vi "CfgManager.Text--ForceSave.vi"() -> ()   [LabVIEW 2013]
uses:
  source/Manager.Text/ConfigManager.Text.lvclass
  source/Manager/Decompose KVPs.vi
  source/Manager/Write.vi
  source/Manager/ConfigManager.lvclass
panel:
  out "Keys":string[](array[string])
  out "error out":errorcluster
  out "filepath":path
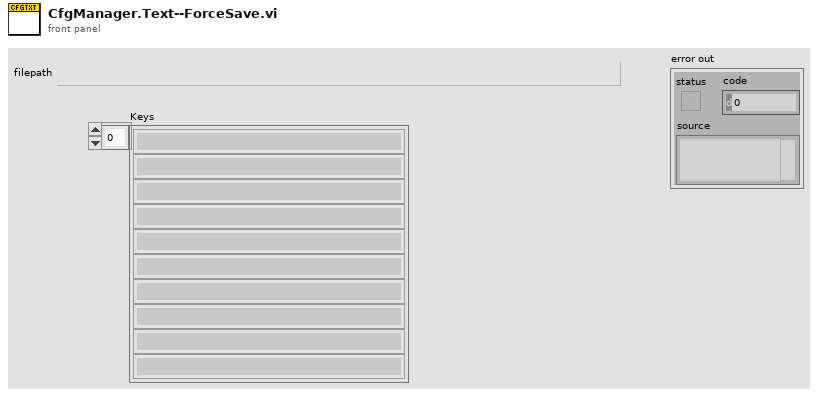
[diagram p1: front panel]
types:
  T1 = cluster{"String":string, "Numeric":dbl, "Boolean":bool}
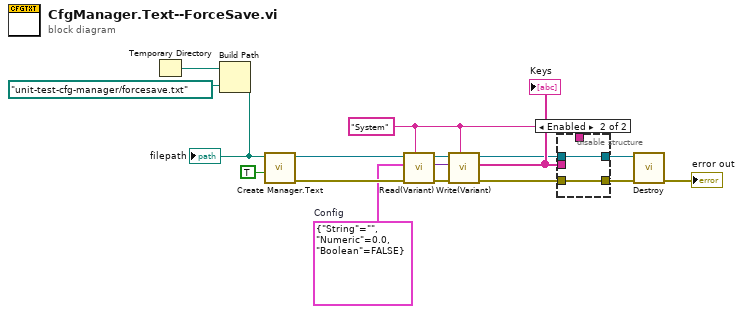
[diagram p0: block diagram]
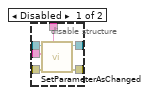
[diagram p2: hidden frame]
diagram:
  w5 = "System" ("Qualified Name")
  w10 = T1 {"String"="", "Numeric"=0.0, "Boolean"=FALSE}  # Config
  n1 = Temporary Directory() -> (w16:path)
  n2 = Build Path(base path=w16, name or relative path=path "unit-test-cfg-manager/forcesave.txt" ("filepath 2")) -> (appended path=w14:path)
  "filepath" <- w14
  n3 = call "Create Manager.Text.vi"("Create if Non Existent? (T)"=TRUE, "filepath"=w14) -> ("error out"=w11:errorcluster, "ConfigManager.Text out"=w12:refnum<class "ConfigManager.Text.lvclass">)  [unwired: 7 in, 1 out]
  n4 = call "Read(Variant).vi"("Qualified Name"=w5, "error in (no error)"=w11, "Type"=w10, "ConfigManager in"=w12) -> ("error out"=w6:errorcluster, "value"=w4:variant, "ConfigManager out"=w7:refnum<class "ConfigManager.Text.lvclass">)  [unwired: 3 in, 2 out]
  n5 = call "Write(Variant).vi"("Qualified Name"=w5, "error in (no error)"=w6, "value"=w4, "ConfigManager in"=w7) -> ("error out"=w1:errorcluster, "keys written"=w3:string[], "ConfigManager out"=w2:refnum<class "ConfigManager.Text.lvclass">)  [unwired: 5 in]
  "Keys" <- w3
  n6 = disable-structure shown="Enabled" {
    disable-tunnel: [w23 w24] -> w9
    disable-tunnel: [w22 w25] -> w8
    disable-tunnel: w5 -> [w21 _]
    disable-tunnel: w3 -> [w20 _]
    disable-tunnel: w2 -> [w19 w25]
    disable-tunnel: w1 -> [w18 w24]
    frame Disabled {
      n7 = call "SetParameterAsChanged.vi"("Qualified Name"=w21, "error in (no error)"=w18, "Keys"=w20, "ConfigManager in"=w19) -> ("error out"=w23:errorcluster, "ConfigManager out"=w22:refnum<class "ConfigManager.Text.lvclass">)  [unwired: 6 in]
    }
    frame Enabled {
    }
  }
  n8 = call-dynamic "Destroy.vi"("error in (no error)"=w9, "ConfigManager.Text in"=w8) -> ("error out"=→"error out":errorcluster)  [unwired: 8 in, 1 out]
